vi "PostStop - Shearbox (SubVI).vi"(8 "error in (no error)":errorcluster, 11 "Cluster in in":T1 {"M Event" items=["Stop", "Running", "PID", "Up Limit", "Down Limit", "Load Limit"]; "Test Type" items=["Please Select", "Triaxial Shear", "Triaxial UU", "Shearbox", "Permeability", "Consolidation (Stepped Loading)/Swelling", "Saturation (Incremental)", "User Defined", "UCT", "Isotropic Consolidation", "Swelling Pressure"]; "Data"."Test Type" items=["Please Select", "Triaxial Shear", "Triaxial UU", "Shearbox", "Permeability", "Consolidation (Stepped Loading)/Swelling", "Saturation (Incremental)", "User Defined", "UCT", "Isotropic Consolidation", "Swelling Pressure"]}) -> (0 "error out":errorcluster, 2 "Enum":T10, 3 "Cluster out":T1 {"M Event" items=["Stop", "Running", "PID", "Up Limit", "Down Limit", "Load Limit"]; "Test Type" items=["Please Select", "Triaxial Shear", "Triaxial UU", "Shearbox", "Permeability", "Consolidation (Stepped Loading)/Swelling", "Saturation (Incremental)", "User Defined", "UCT", "Isotropic Consolidation", "Swelling Pressure"]; "Data"."Test Type" items=["Please Select", "Triaxial Shear", "Triaxial UU", "Shearbox", "Permeability", "Consolidation (Stepped Loading)/Swelling", "Saturation (Incremental)", "User Defined", "UCT", "Isotropic Consolidation", "Swelling Pressure"]})   [LabVIEW 2019]
uses:
  Controls/RunTest - State.ctl
  Controls/RunTest - Data Structure.ctl
  Controls/Test Panel - Data Structure.ctl
  Controls/Station - Test Type.ctl
  <vilib>/Utility/miscctls.llb/LVRowAndColumnTypeDef.ctl
  Controls/RunTest - Calculate Data.ctl
  <vilib>/httpClient/ClientHandle.ctl
  Controls/RunTest - Start Condition.ctl
  Controls/RunTest - Stop Condition.ctl
  Controls/UDP - Event.ctl
  Controls/UDP - Command.ctl
  <vilib>/httpClient/LabVIEWHTTPClient.lvlib
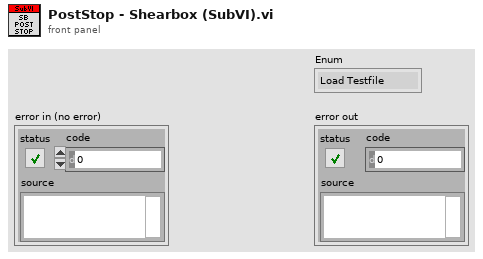
[diagram p1: front panel]
types:
  T1 = typedef "RunTest - Data Structure.ctl" = cluster{"Test Plan":string[], "PlanRow":i32, "Device Name":string[], "Timeout":i32, "Start?":bool, "Pause?":bool, "IP Address":string[], "LogRow":i32, "Logtype":u16, "Log Elapse":sgl, "Data":T2, "Stop log?":bool, "tdms":refnum<k34>, "Sensor Data":sgl[], "Start time":timestamp, "Prev Log Elapse":u32, "Plot":u16, "X-Axis":u16[], "Y-Axis":u16[], "XY":cluster{"X":dbl, "Y":dbl}[][], "End Stage?":bool, "1run":bool, "Condition":u16[], "Start Con":bool, "Log Con":bool, "Stop Con":bool, "Start Elapse":dbl, "Start Load":dbl, "Motor":i32, "StartRow":i32, "number log":i32, "Dir":bool, "Start time test":timestamp, "Auto":bool, "Check return?":bool, "Inv":cluster{"M":i32[], "Bool":bool[]}, "tdms temp":refnum<k34>, "Zero?":bool, "Plot Timer":dbl, "1st Run":bool, "TDMS Path":path, "MaxLoad":dbl, "Log Timer":sgl[], "Test Type":T3, "Log Sensor":string[], "Save?":bool, "1st Log":bool, "Y-Axis 2":u16[], "On Y-Axis 2":bool, "Decimal":u8[], "Init":cluster{"PWP TS":sgl, "Load TS":sgl, "Volume TS":sgl, "Disp TS":sgl, "CP":sgl, "Vol In":sgl, "Vol Out":sgl, "Load UCT":sgl, "Disp UCT":sgl, "PWP Sat":sgl, "CP Sat":sgl, "Volume IsoCons":sgl, "PWP IsoCons":sgl, "PWP TUU":sgl, "Load TUU":sgl, "Volume TUU":sgl, "Disp TUU":sgl, "Load Cons":sgl, "Disp Cons":sgl, "Volume Sat":sgl, "Vertical Load SB":sgl, "Vertical Disp SB":sgl, "H Disp SB":sgl, "H Load SB":sgl}, "Calc":T5, "Device Index":i32[], "Channel Index":i32[], "http ref":T6, "fileid":string, "Step Cons":cluster{"V Stress":sgl, "H Settlement":sgl}, "RunTest":bool, "Graph Last":i32, "Init?":bool, "Datalog":bool[], "Start":T7, "Stop":T8, "Running?":bool, "StartTime":dbl, "Log Prev Time":dbl, "KeyName":string[], "Test RunTime":dbl, "Log Prev Axial":dbl, "M Event":T9[], "Last Log":bool, "popup":bool, "PreStart UU":bool, "PreStart Sat":bool}
  T2 = typedef "Test Panel - Data Structure.ctl" = cluster{"Station":string, "Sample ID":string, "Job No":string, "Job Description":string, "Filename":string, "Test Type":T3, "Speciment No":string, "Depth":string, "Height":string, "Diameter/Length":string, "Weight":string, "Test Parameter":string, "Station[]":string[], "Edit Pos":T4, "Edit Pos Prev":T4, "Area":string, "Path":string}
  T3 = typedef "Station - Test Type.ctl" = u16
  T4 = typedef "LVRowAndColumnTypeDef.ctl" = cluster{"Row":i32, "Column":i32}
  T5 = typedef "RunTest - Calculate Data.ctl" = cluster{"TS":cluster{"Change PWP":sgl, "Change Vol":sgl, "Axial Load":sgl, "CiL":sgl, "Deviator":sgl, "Axial Strain":sgl, "MaxDeviator":sgl}, "TUU":cluster{"Change PWP":sgl, "Axial Load":sgl, "CiL":sgl, "Deviator":sgl, "Axial Strain":sgl, "MaxDeviator":sgl}, "Sat":cluster{"B Value":sgl, "PWP Diss":sgl, "CPP":sgl, "CV":sgl}, "Per":cluster{"Change Vol In":sgl, "Change Vol Out":sgl, "Mean Vol":sgl, "Gradient Pressure":sgl, "Outlet Flow":sgl, "Inlet Flow":sgl, "I X1":sgl, "I X2":sgl, "I Y1":sgl, "I Y2":sgl, "O X1":sgl, "O X2":sgl, "O Y1":sgl, "O Y2":sgl}, "Step Cons":cluster{"V Stress":sgl, "H Settlement":sgl, "Total H Settle":sgl, "Prev Total H":sgl}, "UCT":cluster{"ALC":sgl, "H Change":sgl, "Deviator":sgl, "Axial Strain":sgl, "V Stress":sgl, "MaxDeviator":sgl}, "ISO Cons":cluster{"CPP":sgl, "PWP Diss":sgl, "CV":sgl}, "SB":cluster{"Speci LenC":sgl, "Shear Strain":sgl, "H LC":sgl, "Normal Stress":sgl, "Shear Stress":sgl, "MaxShear":sgl}}
  T6 = typedef "LabVIEWHTTPClient.lvlib/ClientHandle.ctl" = refnum<k1>
  T7 = typedef "RunTest - Start Condition.ctl" = cluster{"Cons":cluster{"VS":dbl, "Delay":bool, "No Delay":dbl}, "Sat":cluster{"CP":dbl, "BP":dbl, "StartBP":bool, "Target CP":bool, "Target BP":bool}, "Iso":cluster{"BP":dbl}, "TS":cluster{"SS":dbl, "Engage":bool, "ES":dbl, "LC":dbl, "PreStart":bool, "Trig SS":bool, "Drain":dbl}, "TUU":cluster{"SS":dbl, "Engage":bool, "ES":dbl, "LC":dbl, "PreStart":bool, "Trig SS":bool, "CP":dbl, "Delay Value":dbl, "Delay":bool, "CP PID":bool}, "UCT":cluster{"SS":dbl, "Engage":bool, "ES":dbl, "LC":dbl, "PreStart":bool, "Trig SS":bool}, "Enable?":bool, "SB":cluster{"SS":dbl, "Engage":bool, "ES":dbl, "LC":dbl, "PreStart":bool, "Trig SS":bool, "VS":dbl, "Delay Value":dbl, "Delay":bool, "VS PID":bool}, "Perm":cluster{"DP":dbl}}
  T8 = typedef "RunTest - Stop Condition.ctl" = cluster{"Cons":cluster{"Select":i32, "Disp":dbl, "Time":dbl, "Time2":dbl, "Disp 2":dbl, "Time Cond":dbl, "Last Disp":dbl, "Swell":bool}, "Sat":cluster{"Select":i32, "PP":dbl, "Time":dbl, "VC":dbl, "Time2":dbl, "Time Cond":dbl, "Last PP":dbl, ".B":bool, "B":dbl, "Last Vc":dbl, "Time Cond 2":dbl, "Time3":dbl, "Time Cond 3":dbl}, "Iso":cluster{"PP":dbl, "Time":dbl, "VC":dbl, "Time2":dbl, "Time Cond":dbl, "Last Vc":dbl, ".PP":bool, "Time Cond 2":dbl, "Select":i32}, "TS":cluster{"Axial":dbl, ".MaxDev":bool, "MaxDev Value":dbl, "Return":bool, "Reset":bool, "Prev Time":dbl, "PostStop Run":bool, "CP Stop":bool, "BP Stop":bool, "PostStop Trig":bool, "Reset Value":dbl, "BPTrig":bool, "CPTrig":bool, "VLCTrig":bool}, "TUU":cluster{"Axial":dbl, ".MaxDev":bool, "MaxDev Value":dbl, "Return":bool, "Reset":bool, "Prev Time":dbl, "PostStop Run":bool, "CP Stop":bool, "BP Stop":bool, "PostStop Trig":bool, "Reset Value":dbl, "BPTrig":bool, "CPTrig":bool, "VLCTrig":bool}, "UCT":cluster{"Axial":dbl, ".MaxDev":bool, "MaxDev Value":dbl, "Return":bool, "Reset":bool, "Prev Time":dbl, "PostStop Run":bool, "CP Stop":bool, "BP Stop":bool, "PostStop Trig":bool}, "Enable?":bool, "SB":cluster{"Shear":dbl, ".MaxShear":bool, "MaxShear Value":dbl, "Return":bool, "Reset":bool, "Prev Time":dbl, "PostStop Run":bool, "CP Stop":bool, "BP Stop":bool, "PostStop Trig":bool, "Reset Value":dbl, "BPTrig":bool, "CPTrig":bool, "VLCTrig":bool}, "Perm":cluster{"Max Time":bool, "Reset":bool, "PostStop Run":bool, "Ratio":bool, "Reset Value":dbl, "Time":dbl, "RatioTime":dbl, "RatioMore":dbl, "RatioLess":dbl, "Time Cond":dbl, "Time Cond 2":dbl, "Prev IF":dbl, "Prev OF":dbl, "PostStop Trig":bool, "BP Trig":bool, "DP Stop":bool, "BP Stop":bool, "CP Stop":bool, "CP Trig":bool}, "SP":cluster{".Max Time":bool, ".Time":bool, "Time":dbl, "MaxTime":dbl, "Time Cond":dbl, "Max Time Cond":dbl, "Stress":dbl}}
  T9 = typedef "UDP - Event.ctl" = u16
  T10 = typedef "RunTest - State.ctl" = enum16{"Load Testfile", "Notifier", "Init", "Idle", "Load", "Read DB", "Run", "Pause", "Stop", "Check Start", "Check Stop", "Check Post Stop", "Check Log", "EndStage", "Data View", "Display", "Graph", "Graph Old", "Close", "Stop PID", "Check Limit", "Auto", "Up", "Log", "Zero", "Machine Control", "Save Report"}
  T11 = enum32{"Please Select", "Triaxial Shear", "Triaxial UU", "Shearbox", "Permeability", "Consolidation", "Saturation", "User Defined", "UCT", "Iso Consolidation"}
  T12 = typedef "UDP - Command.ctl" = enum16{"Stop", "Jog Up", "Jog Down", "Ramp Up", "Ramp Down", "PID Target", "PID Ramp", "Disp Run", "Read Ch Data", "Zero Channel", "Zero Disp", "Read Sensor", "Write Sensor", "Read ADC", "Write ADC", "Read PID", "Write PID", "Read Test", "Write Test", "Read System", "Write System", "Read Datalog", "Read Datalog Sensor"}
  T13 = cluster{"Target Load":sgl, "Target Disp":sgl, "Rate":sgl, "Speed":sgl}
  T14 = enum16{"None", "Run Target", "Run Ramp", "Run Disp"}
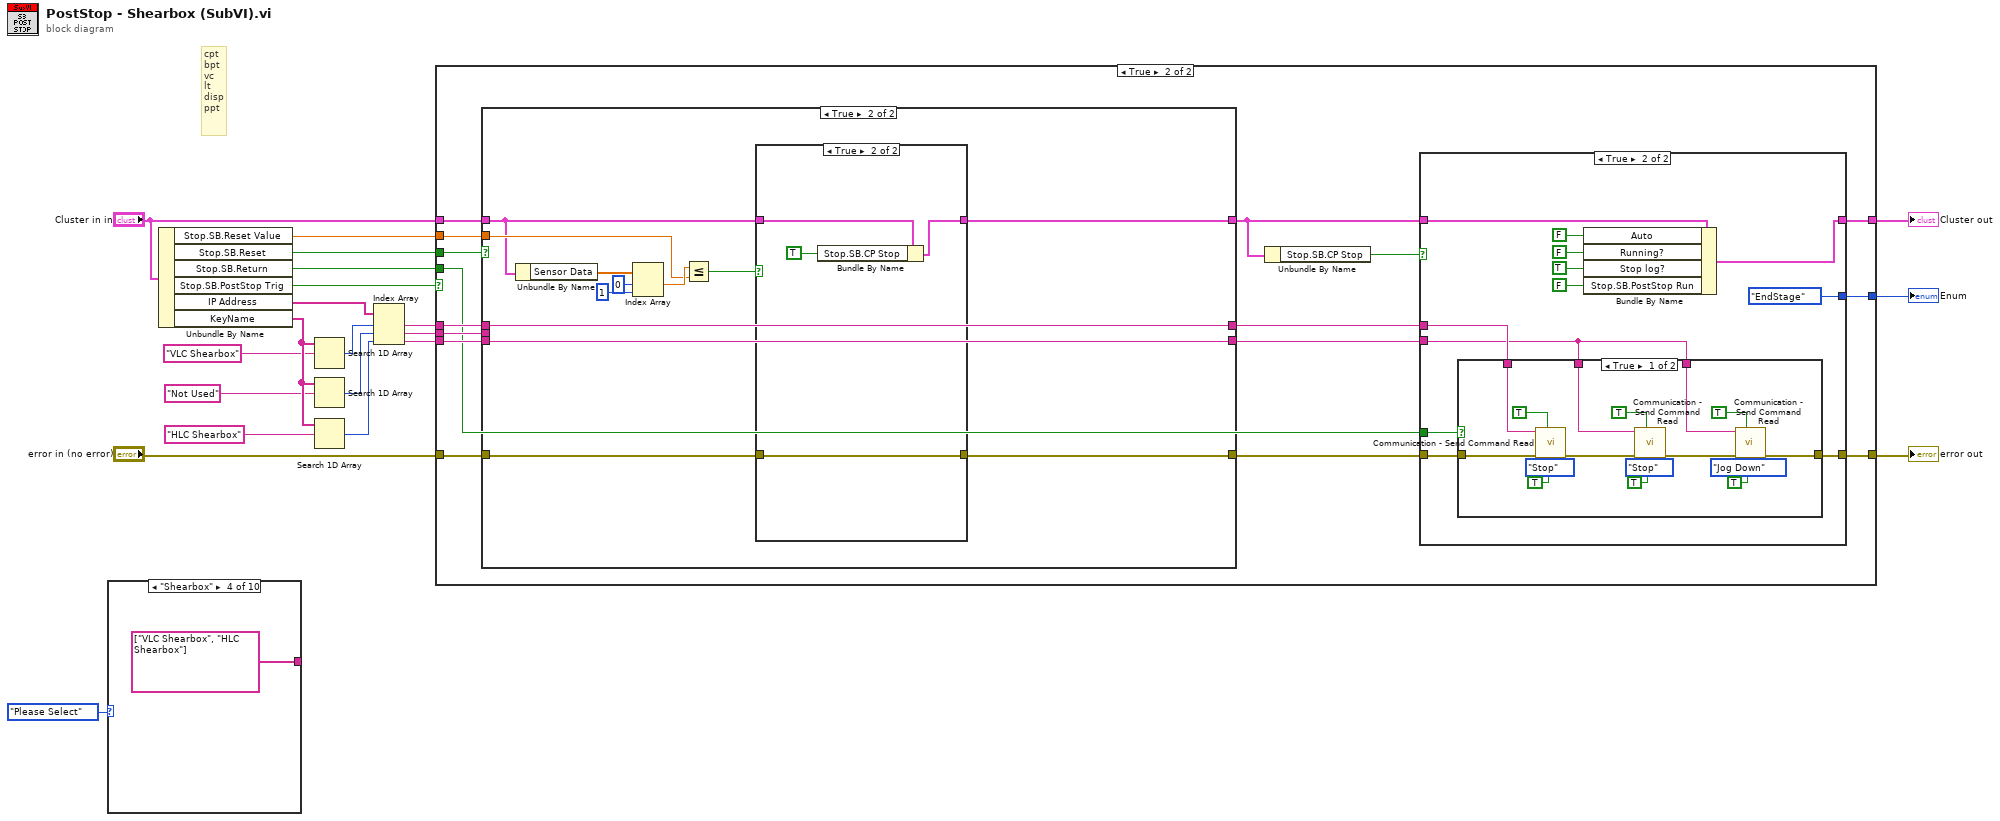
[diagram p0: block diagram]
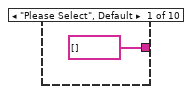
[diagram p2: hidden frame]
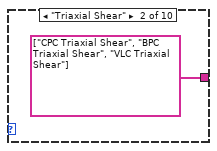
[diagram p3: hidden frame]
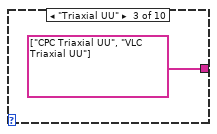
[diagram p4: hidden frame]
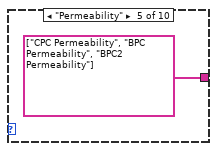
[diagram p5: hidden frame]
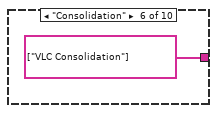
[diagram p6: hidden frame]
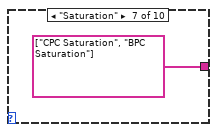
[diagram p7: hidden frame]
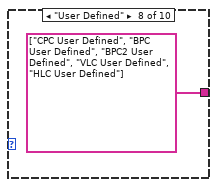
[diagram p8: hidden frame]
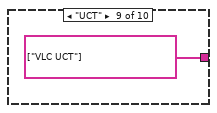
[diagram p9: hidden frame]
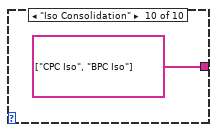
[diagram p10: hidden frame]
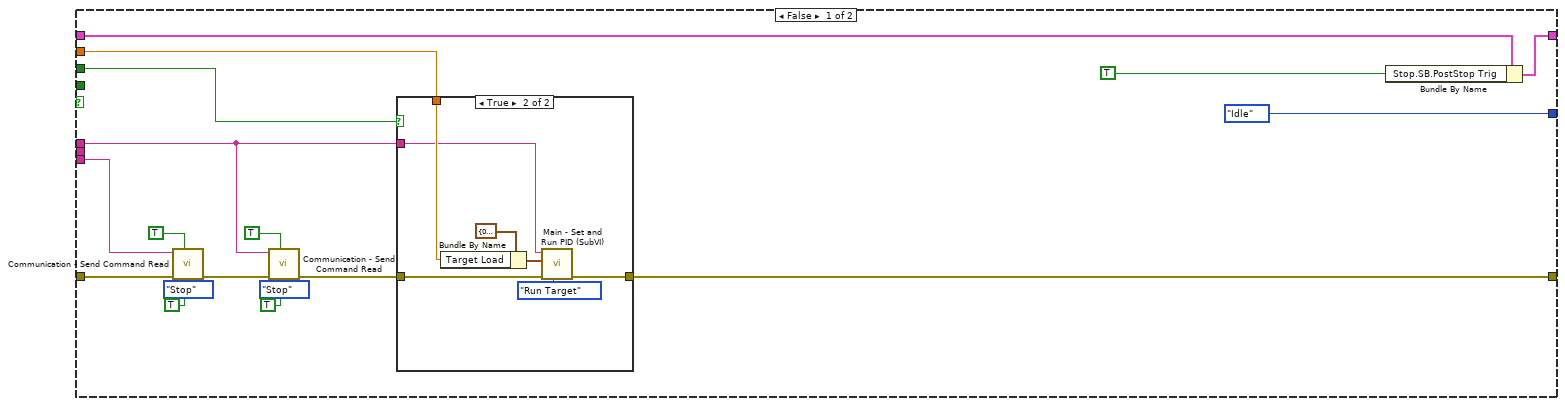
[diagram p11: hidden frame]
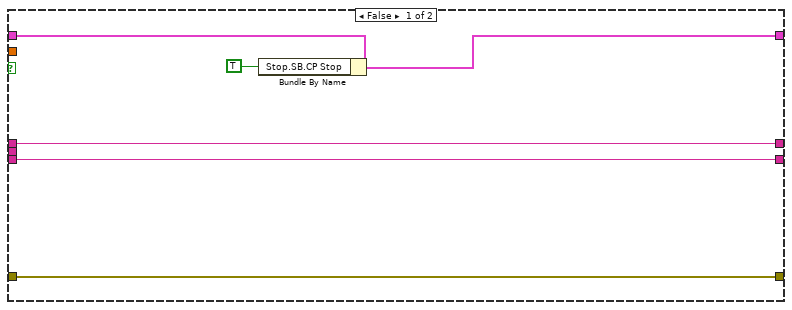
[diagram p13: hidden frame]
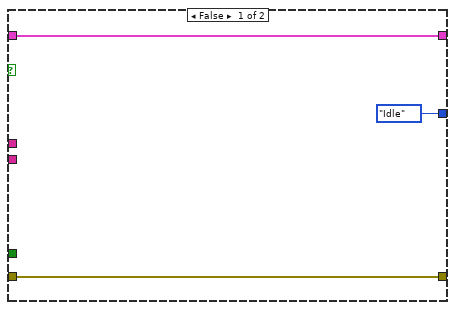
[diagram p15: hidden frame]
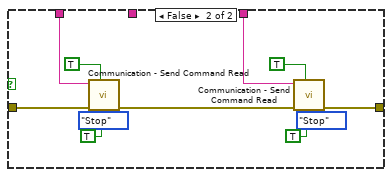
[diagram p16: hidden frame]
diagram:
  # "cpt\nbpt\nvc\nlt\ndisp\nppt"
  n1 = case shown="\"Shearbox\"" T11."Please Select" ("Sub Tab") {
    tunnel: [string[] [] string[] ["CPC Triaxial Shear", "BPC Triaxial Shear", "VLC Triaxial Shear"] string[] ["CPC Triaxial UU", "VLC Triaxial UU"] string[] ["VLC Shearbox", "HLC Shearbox"] string[] ["CPC Permeability", "BPC Permeability", "BPC2 Permeability"] string[] ["VLC Consolidation"] string[] ["CPC Saturation", "BPC Saturation"] string[] ["CPC User Defined", "BPC User Defined", "BPC2 User Defined", "VLC User Defined", "HLC User Defined"] string[] ["VLC UCT"] string[] ["CPC Iso", "BPC Iso"]] -> _
    frame "Please Select", Default {
    }
    frame "Triaxial Shear" {
    }
    frame "Triaxial UU" {
    }
    frame "Shearbox" {
    }
    frame "Permeability" {
    }
    frame "Consolidation" {
    }
    frame "Saturation" {
    }
    frame "User Defined" {
    }
    frame "UCT" {
    }
    frame "Iso Consolidation" {
    }
  }
  n2 = Unbundle By Name("Cluster in in") -> ("Stop.SB.Reset Value"=w21:dbl, "Stop.SB.Reset"=w19:bool, "Stop.SB.Return"=w18:bool, "Stop.SB.PostStop Trig"=w3:bool, "IP Address"=w20:string[], "KeyName"=w16:string[])
  n3 = Search 1D Array(1D array=w16, element="VLC Shearbox" ("String")) -> (index of element=w9:i32)  [unwired: 1 in]
  n4 = Search 1D Array(1D array=w16, element="Not Used" ("String")) -> (index of element=w10:i32)  [unwired: 1 in]
  n5 = Search 1D Array(1D array=w16, element="HLC Shearbox" ("String")) -> (index of element=w15:i32)  [unwired: 1 in]
  n6 = Index Array(array=w20, index #1=w9, index #2=w10, index #3=w15) -> (element #1=w11:string, element #2=w12:string, element #3=w17:string)
  n7 = case shown="True" w3 {
    tunnel: [w47 w68] -> w4
    tunnel: "Cluster in in" -> [w49 w69]
    tunnel: [w38 w66] -> w6
    tunnel: "error in (no error)" -> [w41 w73]
    tunnel: w11 -> [w32 w72]
    tunnel: w12 -> [_ w71]
    tunnel: [RunTest_-_State."Idle" w70] -> w13
    tunnel: w17 -> [w40 w62]
    tunnel: w18 -> [_ w60]
    tunnel: w19 -> [w45 w58]
    tunnel: w21 -> [w39 w64]
    frame False {
      n8 = call "Communication - Send Command Read.vi"("Fron?"=TRUE, "Bypass?"=TRUE, "error in (no error)"=w41, "Action"=UDP_-_Command."Stop", "Device IP Address"=w40) -> ("error out"=w34:errorcluster)  [unwired: 6 in]
      n9 = call "Communication - Send Command Read.vi"("Fron?"=TRUE, "Bypass?"=TRUE, "error in (no error)"=w34, "Action"=UDP_-_Command."Stop", "Device IP Address"=w32) -> ("error out"=w33:errorcluster)  [unwired: 6 in]
      n10 = case shown="True" w45 {
        tunnel: w33 -> [w50 w54]
        tunnel: w32 -> [_ w51]
        tunnel: [w50 w52] -> w38
        tunnel: w39 -> [_ w53]
        frame False {
        }
        frame True {
          n11 = Bundle By Name(cluster=T13 {"Target Load"=0.0, "Target Disp"=0.0, "Rate"=0.0, "Speed"=0.0} ("Test"), "Target Load"=w53) -> (w55:T13)
          n12 = call "Main - Set and Run PID (SubVI).vi"("Action"=T14."Run Target", "error in (no error)"=w54, "Test"=w55, "IP Address"=w51) -> ("error out"=w52:errorcluster)  [unwired: 7 in]
        }
      }
      n13 = Bundle By Name(cluster=w49, "Stop.SB.PostStop Trig"=TRUE ("Stop.TS.PostStop Run")) -> (w47:T1)
    }
    frame True {
      n14 = case shown="True" w58 {
        tunnel: w73 -> [w76 w80]
        tunnel: w72 -> [w75 w83]
        tunnel: w71 -> [_ _]
        tunnel: w69 -> [w78 w81]
        tunnel: [w77 w91] -> w67
        tunnel: [w76 w90] -> w65
        tunnel: w64 -> [_ w84]
        tunnel: [w75 w83] -> w63
        tunnel: w62 -> [w74 w82]
        tunnel: [w74 w82] -> w61
        frame False {
          n15 = Bundle By Name(cluster=w78, "Stop.SB.CP Stop"=TRUE ("Stop.TS.CP Stop")) -> (w77:T1)
        }
        frame True {
          n16 = Unbundle By Name(w81) -> ("Sensor Data"=w89:sgl[])
          n17 = Index Array(array=w89, index #1=0 ("index"), index #2=1 ("index")) -> (element #1=w86:sgl)  [unwired: 1 out]
          n18 = Less Or Equal?(x=w86, y=w84) -> (x <= y?=w85:bool)
          n19 = case shown="True" w85 {
            tunnel: w80 -> [w93 w94]
            tunnel: [w93 w94] -> w90
            tunnel: w81 -> [w92 w96]
            tunnel: [w92 w95] -> w91
            frame False {
            }
            frame True {
              n20 = Bundle By Name(cluster=w96, "Stop.SB.CP Stop"=TRUE ("Stop.TS.BP Stop")) -> (w95:T1)
            }
          }
        }
      }
      n21 = Unbundle By Name(w67) -> ("Stop.SB.CP Stop"=w59:bool)
      n22 = case shown="True" w59 {
        tunnel: [RunTest_-_State."Idle" RunTest_-_State."EndStage"] -> w70
        tunnel: [w99 w109] -> w68
        tunnel: w67 -> [w99 w111]
        tunnel: [w98 w104] -> w66
        tunnel: w65 -> [w98 w106]
        tunnel: w63 -> [_ w105]
        tunnel: w61 -> [_ w101]
        tunnel: w60 -> [_ w103]
        frame False {
        }
        frame True {
          n23 = case shown="True" w103 {
            tunnel: w106 -> [w120 w131]
            tunnel: w105 -> [w114 w129]
            tunnel: [w122 w133] -> w104
            tunnel: w101 -> [w121 w132]
            tunnel: w101 -> [w113 _]
            frame True {
              n24 = call "Communication - Send Command Read.vi"("Fron?"=TRUE, "Bypass?"=TRUE, "error in (no error)"=w120, "Action"=UDP_-_Command."Stop", "Device IP Address"=w114) -> ("error out"=w116:errorcluster)  [unwired: 6 in]
              n25 = call "Communication - Send Command Read.vi"("Fron?"=TRUE, "Bypass?"=TRUE, "error in (no error)"=w116, "Action"=UDP_-_Command."Stop", "Device IP Address"=w113) -> ("error out"=w115:errorcluster)  [unwired: 6 in]
              n26 = call "Communication - Send Command Read.vi"("Fron?"=TRUE, "Bypass?"=TRUE, "error in (no error)"=w115, "Action"=UDP_-_Command."Jog Down", "Device IP Address"=w121) -> ("error out"=w122:errorcluster)  [unwired: 6 in]
            }
            frame False {
              n27 = call "Communication - Send Command Read.vi"("Fron?"=TRUE, "Bypass?"=TRUE, "error in (no error)"=w131, "Action"=UDP_-_Command."Stop", "Device IP Address"=w129) -> ("error out"=w130:errorcluster)  [unwired: 6 in]
              n28 = call "Communication - Send Command Read.vi"("Fron?"=TRUE, "Bypass?"=TRUE, "error in (no error)"=w130, "Action"=UDP_-_Command."Stop", "Device IP Address"=w132) -> ("error out"=w133:errorcluster)  [unwired: 6 in]
            }
          }
          n29 = Bundle By Name(cluster=w111, "Auto"=FALSE, "Running?"=FALSE, "Stop log?"=TRUE, "Stop.SB.PostStop Run"=FALSE ("Stop.TUU.PostStop Run")) -> (w109:T1)
        }
      }
    }
  }
  "Enum" <- w13
  "error out" <- w6
  "Cluster out" <- w4
